vi "Cluster to Array of Variants.vi"(8 "error in (no error)":errorcluster, 11 "Section (Cluster)":variant) -> (0 "error out":errorcluster, 2 "Cluster Elements":variant[](array[variant]), 3 "Section (Cluster) out":variant)   [LabVIEW 2020, in "Generic Config Handling.lvlib"]
doc: "This vi takes a cluster that has been converted to a variant and extracts all of its elements and converts them into variants and returns an array of variants."
uses:
  Generic Config Handling.lvlib
  <vilib>/Utility/VariantDataType/Type.ctl
  <vilib>/Utility/VariantDataType/VariantType.lvlib
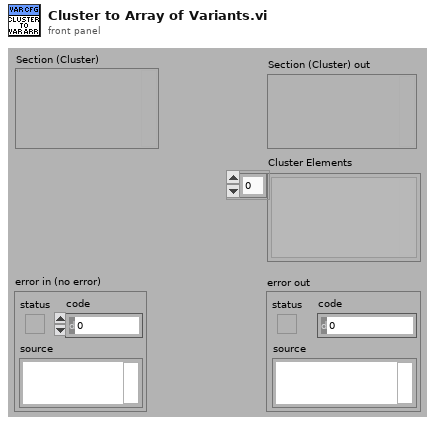
[diagram p1: front panel]
types:
  T1 = typedef "VariantType.lvlib/Type.ctl" = enum8{"Invalid Type", "Void", "I8", "I16", "I32", "I64", "U8", "U16", "U32", "U64", "Single Float", "Double Float", "Extended Float", "Single Complex", "Double Complex", "Extended Complex", "Enum U8", "Enum U16", "Enum U32", "Enum U64", "Single Float With Unit", "Double Float With Unit", "Extended Float With Unit", "Single Complex with Unit", "Double Complex with Unit", "Extended Complex with Unit", "Boolean", "String", "Path", "Picture", "Tag", "Array", "Cluster", "Variant", "LV Variant", "Waveform", "Timestamp", "Digital Waveform", "Digital Data", "ExpressData", "Refnum", "External Data", "VI", "Poly VI", "LabVIEW Class Instance", "Fixed Point"}
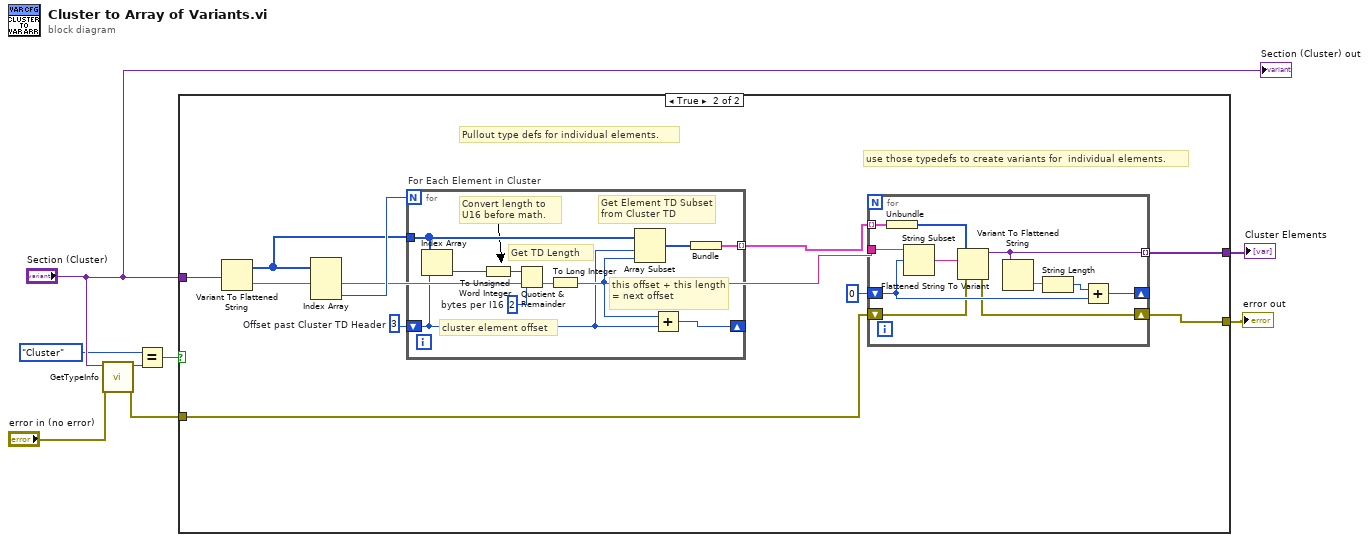
[diagram p0: block diagram]
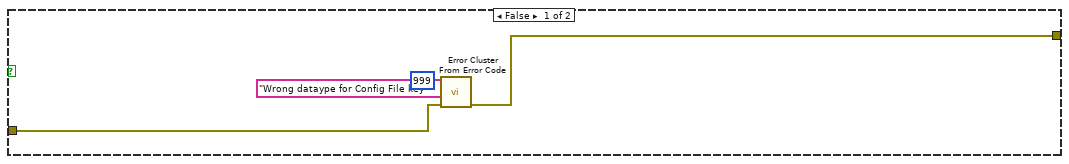
[diagram p2: hidden frame]
diagram:
  n1 = call <vilib>:"GetTypeInfo.vi"("error in (no error)"="error in (no error)", "Variant"="Section (Cluster)") -> ("error out"=w3:errorcluster, "Type Enum"=w7:T1)  [unwired: 5 in, 3 out]
  n2 = Equal?(x=Type."Cluster" ("Type Enum"), y=w7) -> (x = y?=w5:bool)
  n3 = case shown="True" w5 {
    tunnel: "Section (Cluster)" -> [_ w14]
    tunnel: w3 -> [w11 w13]
    tunnel: [_ w16] -> w2
    tunnel: [w10 w17] -> w1
    frame False {
      n4 = call <vilib>:"Error Cluster From Error Code.vi"("error in (no error)"=w11, "error message (\"\")"="Wrong dataype for Config File key" ("error message (\"\")"), "error code (0)"=999) -> ("error out"=w10:errorcluster)  [unwired: 6 in]
    }
    frame True {
      w22 = 3  # Offset past Cluster TD Header
      # "use those typedefs to create variants for  individual elements."
      # "Pullout type defs for individual elements."
      n5 = Variant To Flattened String(Variant=w14) -> (data string=w18:string, 1:w20:i16[])
      n6 = Index Array(array=w20) -> (element #3=w21:i16)  [unwired: 3 in, 2 out]
      n7 = for "For Each Element in Cluster" {
        N: w21 -> [_]
        shift-right: [w41] -> _
        shift-left: w22 -> [w40]
        tunnel: w20 -> [w42]
        tunnel: [w36] -> w19 mode=indexing
        w37 = u16 2  # bytes per I16
        # "Get TD Length"
        # "this offset + this length = next offset"
        # "cluster element offset"
        # "Get Element TD Subset from Cluster TD"
        # "Convert length to U16 before math."
        n8 = Index Array(array=w42, index=w40) -> (element=w38:i16)
        n9 = To Unsigned Word Integer(number=w38) -> (unsigned 16bit integer=w35:u16)
        n10 = Quotient & Remainder(x=w35, y=w37) -> (floor(x/y)=w39:u16)  [unwired: 1 out]
        n11 = To Long Integer(number=w39) -> (32bit integer=w34:i32)
        n12 = Array Subset(array=w42, index=w40, length=w34) -> (w43:i16[])
        n13 = Add(x=w34, y=w40) -> (x+y=w41:i32)
        n14 = Bundle(w43) -> (w36:cluster{i16[]})  [unwired: 1 in]
      }
      n15 = for {
        tunnel: w18 -> [w30]
        tunnel: [w33] -> w16 mode=indexing
        shift-right: [w27] -> _
        shift-left: 0 -> [w29]
        shift-right: [w25] -> w17
        shift-left: w13 -> [w26]
        tunnel: w19 -> [w24] mode=indexing
        n16 = Unbundle(w24) -> (w23:i16[])
        n17 = String Subset(string=w30, offset (0)=w29) -> (substring=w31:string)  [unwired: 1 in]
        n18 = Flattened String To Variant(4:w26, 6:w31, 7:w23) -> (0:w25:errorcluster, 3:w33:variant)
        n19 = Variant To Flattened String(Variant=w33) -> (data string=w32:string)  [unwired: 1 out]
        n20 = String Length(string=w32) -> (length=w28:i32)
        n21 = Add(x=w28, y=w29) -> (x+y=w27:i32)
      }
    }
  }
  "Cluster Elements" <- w2
  "error out" <- w1
  "Section (Cluster) out" <- "Section (Cluster)"
